vi "VI Tree.vi"   [LabVIEW 2012, in "Phidget Digital Input.lvlib"]
doc: "${DigitalInput:VITreeHeader}"
uses:
  <instrlib>/Phidgets/Phidget Digital Input/Phidget Digital Input.lvlib
  <instrlib>/Phidgets/Phidget Digital Input/Public/DigitalInputStart.vi
  <instrlib>/Phidgets/Phidget Digital Input/Public/DigitalInputOpen.vi
  <instrlib>/Phidgets/Phidget Digital Input/Public/DigitalInputClose.vi
panel:
  # "(c) 2015 Phidgets Inc..  ALL RIGHTS RESERVED."
  # "SEE DIAGRAM\nFOR VI TREE."
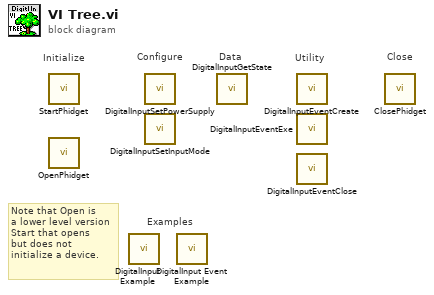
[diagram p0: block diagram]
diagram:
  # "Configure"
  # "Note that Open is\na lower level version\nStart that opens\nbut does not \ninitialize a device."
  # "Examples"
  # "Utility"
  # "Data"
  # "Close"
  # "Initialize"
  n1 = call-poly <instrlib>:"StartPhidget.vi"() -> ()  [unwired: 12 in, 4 out]
  n2 = call-poly <instrlib>:"OpenPhidget.vi"() -> ()  [unwired: 8 in, 4 out]
  n3 = call <instrlib>:"DigitalInput Example.vi"() -> ()  [unwired: 12 in]
  n4 = call <instrlib>:"DigitalInputSetPowerSupply.vi"() -> ()  [unwired: 9 in, 2 out]
  n5 = call <instrlib>:"DigitalInputSetInputMode.vi"() -> ()  [unwired: 9 in, 2 out]
  n6 = call <instrlib>:"DigitalInput Event Example.vi"() -> ()  [unwired: 12 in]
  n7 = call <instrlib>:"DigitalInputGetState.vi"() -> ()  [unwired: 7 in, 4 out]
  n8 = call <instrlib>:"DigitalInputEventCreate.vi"() -> ()  [unwired: 9 in, 3 out]
  n9 = call <instrlib>:"DigitalInputEventExe.vi"() -> ()  [unwired: 4 in, 8 out]
  n10 = call <instrlib>:"DigitalInputEventClose.vi"() -> ()  [unwired: 10 in, 2 out]
  n11 = call-poly <instrlib>:"ClosePhidget.vi"() -> ()  [unwired: 11 in, 1 out]
